vi "Serialize.vi"(8 "error in":errorcluster, 9 "OwningElement in":refnum<k20>, 10 "Document in":refnum<k20>, 11 "FailureReference in":refnum<class "FailureReference.lvclass">) -> (0 "error out":errorcluster, 1 "OwningElement out":refnum<k20>, 2 "Document out":refnum<k20>, 3 "FailureReference out":refnum<class "FailureReference.lvclass">)   [LabVIEW 2021, in "ProligentXMLGenerator.lvlib" / "FailureReference.lvclass"]
uses:
  FailureReference.lvclass
  FailureReference.lvclass/FailureReference.ctl
  <vilib>/xml/NI_XML.lvlib
  Base/DOMSupport/DOMSupport.lvlib
  Model/CustomData/CustomData.lvclass
  <vilib>/xml/Close Reference(Node).vi
  Base/Guid/Guid.lvclass
  C:/Projects/proligent-xml-generator-labview/src/ProligentXMLGenerator/Base/NonEmptyString/NonEmptyString.lvclass
  C:/Projects/proligent-xml-generator-labview/src/ProligentXMLGenerator/Base/String/String.lvclass
  C:/Projects/proligent-xml-generator-labview/src/ProligentXMLGenerator/Base/Attribute/Attribute.lvclass
  C:/Projects/proligent-xml-generator-labview/src/ProligentXMLGenerator/Base/Guid/Guid.lvclass
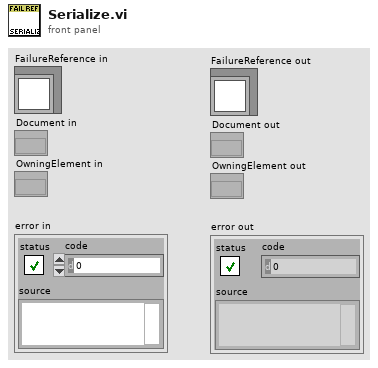
[diagram p1: front panel]
types:
  T1 = typedef "ProligentXMLGenerator.lvlib/FailureReference.lvclass/Data.ctl" = cluster{"Name":string, "CustomData":refnum<class "CustomData.lvclass">, "Id":refnum<class "Guid.lvclass">}
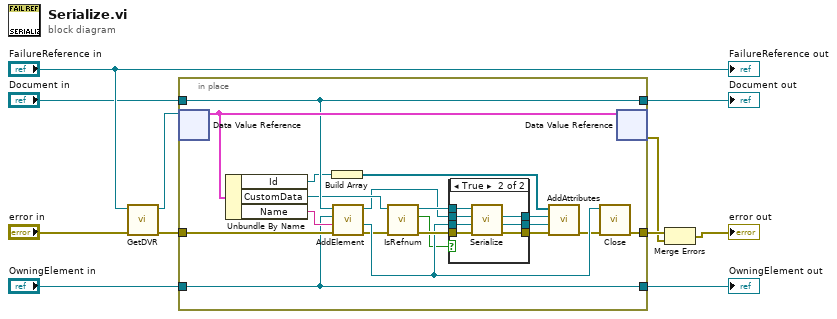
[diagram p0: block diagram]
diagram:
  n1 = call "GetDVR.vi"("error in"="error in", "FailureReference in"="FailureReference in") -> ("error out"=w3:errorcluster, "DVRReference"=w2:refnum<data-value>)  [unwired: 8 in]
  n2 = in-place "In Place Element Structure" {
    in-place-border: [w30] -> w4
    in-place-border: "Document in" -> [w25]
    in-place-border: w3 -> [w29]
    in-place-border: "OwningElement in" -> [w27]
    in-place-border: [w27] -> w6
    in-place-border: [w25] -> w5
    n3 = in-place-dvr #1(w2) -> (w26:T1)  [unwired: 1 out]
    n4 = Unbundle By Name(w26) -> ("Id"=w19:refnum<class "Guid.lvclass">, "CustomData"=w21:refnum<class "CustomData.lvclass">, "Name"=w28:string)
    n5 = Build Array(w19) -> (w18:refnum<class "Guid.lvclass">[])
    n6 = call "AddElement.vi"("error in"=w29, "Name"=w28, "OwningElement in"=w27, "Document in"=w25) -> ("error out"=w13:errorcluster, "NewElement"=w23:refnum<k20>, "Document out"=w17:refnum<k20>)  [unwired: 4 in, 1 out]
    n7 = call "IsRefnum.vi"("error in"=w13, "CustomDataType in"=w21) -> ("error out"=w24:errorcluster, "IsRefnum"=w20:bool, "CustomDataType out"=w22:refnum<class "CustomData.lvclass">)  [unwired: 7 in]
    n8 = case shown="True" w20 {
      tunnel: w17 -> [w32 w40]
      tunnel: w24 -> [w33 w39]
      tunnel: w23 -> [w31 w38]
      tunnel: [w33 w37] -> w14
      tunnel: w22 -> [_ w36]
      tunnel: [w32 w35] -> w15
      tunnel: [w31 w34] -> w16
      frame False {
      }
      frame True {
        n9 = call "Serialize.vi"("error in"=w39, "OwningElement in"=w38, "Document in"=w40, "CustomDataType in"=w36) -> ("error out"=w37:errorcluster, "OwningElement out"=w34:refnum<k20>, "Document out"=w35:refnum<k20>)  [unwired: 4 in, 1 out]
      }
    }
    n10 = call "AddAttributes.vi"("error in"=w14, "OwningElement in"=w16, "Document in"=w15, "Attributes"=w18) -> ("error out"=w12:errorcluster)  [unwired: 5 in, 2 out]
    n11 = call-poly <vilib>:"Close.vi"("error in (no error)"=w12, "node"=w23) -> ("error out"=w30:errorcluster)  [unwired: 7 in]
    n12 = in-place-dvr #1(w26) -> (w1:errorcluster)  [unwired: 1 out]
  }
  "Document out" <- w5
  "OwningElement out" <- w6
  n13 = Merge Errors(w4, w1) -> (→"error out":errorcluster)
  "FailureReference out" <- "FailureReference in"
